vi "re_DataLog Query_srv.vi"(0 "method":T3, 1 "time step":dbl, 5 "begin of range":dbl format="%<%H:%M:%S%2u\n%Y/%m/%d>T", 7 "certificate":string, 9 "end of range":dbl format="%<%H:%M:%S%2u\n%Y/%m/%d>T", 11 "tag":string, 12 "database (current)":string) -> (3 "mode {read range}":T1, 4 "values":dbl[](array[numeric]), 6 "times":dbl[](array[numeric]) format="%<%H:%M:%S%2u\n%Y/%m/%d>T", 8 "points":T2[](array[typedef]) {"value" format="%.3e"; "time" format="%<%H:%M:%S%2u\n%Y/%m/%d>T"}, 10 "strings":string[](array[string]), 15 "error out":errorcluster)   [LabVIEW 2012]
uses:
  typedefs/t_DataLog Query Served Methods.ctl
  typedefs/t_Datalog Datebase Modes.ctl
  typedefs/clusters/t_DataLog Point.ctl
  clientsrv/typedefs/t_ClientSrv Access Levels.ctl
  typedefs/t_DataLog Databases Methods.ctl
  typedefs/t_DataLog Tag Info List Methods.ctl
  subvis/private/glb_DataLog Runtime Parameterisation.vi
panel:
  # "Update panel typedef\nafter changing panel."
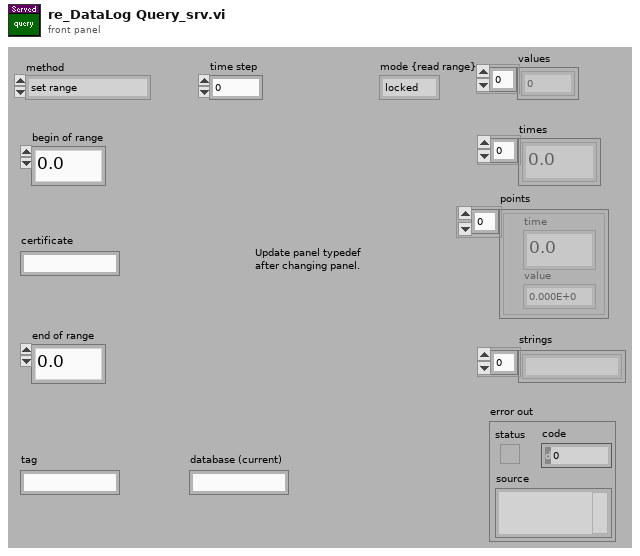
[diagram p1: front panel]
types:
  T1 = typedef "t_Datalog Datebase Modes.ctl" = enum16{"locked", "unlocked", "live", "mirrored"}
  T2 = typedef "t_DataLog Point.ctl" = cluster{"time":dbl, "value":dbl}
  T3 = typedef "t_DataLog Query Served Methods.ctl" = enum16{"set range", "step times", "get times", "interpolate", "interpolate str", "read range", "read str range", "merge&read range", "merge&read str range", "merge range", "clear"}
  T4 = typedef "t_ClientSrv Access Levels.ctl" = enum16{"observer", "operator", "local"}
  T5 = typedef "t_DataLog Tag Info List Methods.ctl" = enum16{"initialize", "create", "create empty", "rename", "delete", "test tag", "get", "get by name", "get default", "get list", "get path", "get subsets", "set subsets", "set config", "set capacity", "#tags", "go live", "set unlocked", "set mirrored"}
  T6 = typedef "t_DataLog Databases Methods.ctl" = enum16{"initialize", "get ref", "get names", "cleanup"}
  T7 = typedef "t_DataLog Database Info Pane.ctl" = refnum<vi>
  T8 = typedef "t_DataLog Tag Config.ctl" = cluster{"name":string, "unit":string, "temporal":T9, "value":T10, "index":i32, "capacity":i32, "is meta?":bool, "mincapacity":i32, "deadband":dbl, "limit delay":dbl, "format":T11, "precision":u8, "undefine":bool, "update":bool, "update period":u16, "expression":string, "description":string, "logging algorithm":T12, "logging parameters":dbl[]}
  T9 = typedef "t_DataLog Temporal Types.ctl" = enum16{"set&hold", "sample", "event"}
  T10 = typedef "t_DataLog Value Types.ctl" = enum16{"number", "string"}
  T11 = typedef "t_DataLog Numerical Format.ctl" = enum8{"fractional", "exponential", "engineering"}
  T12 = typedef "t_DataLog Logging Algorithms.ctl" = enum16{"nothing", "changes", "everything", "every Nth", "time threshold", "value threshold + prior", "t or v threshold", "t or v threshold + prior"}
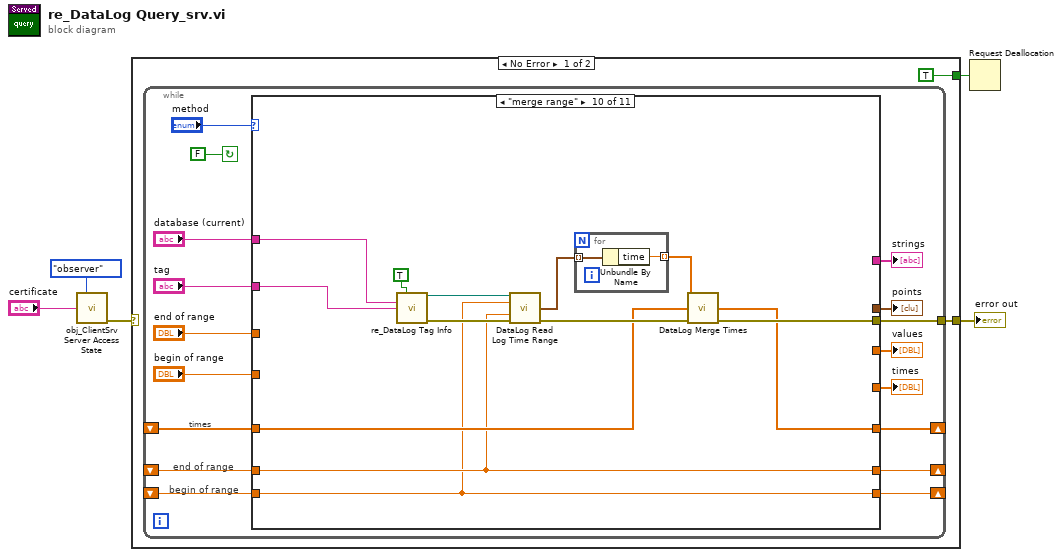
[diagram p0: block diagram]
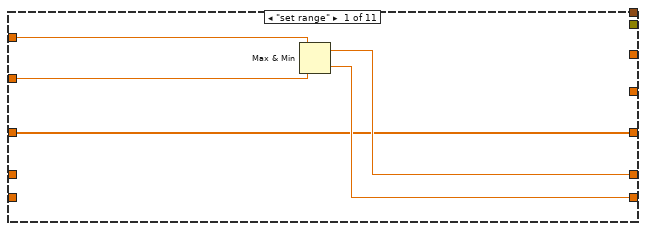
[diagram p2: hidden frame]
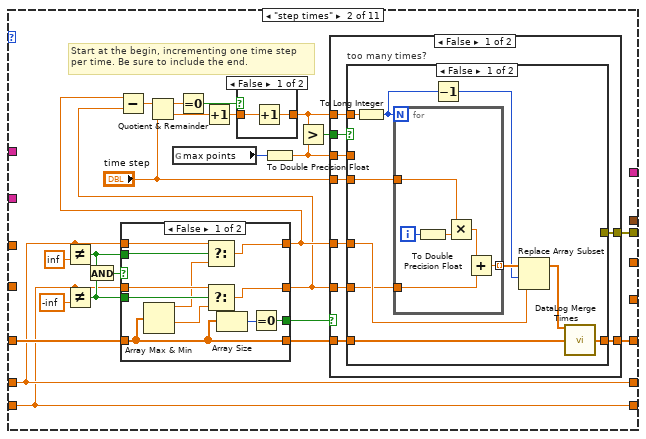
[diagram p3: hidden frame]
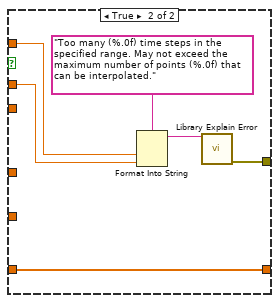
[diagram p4: hidden frame]
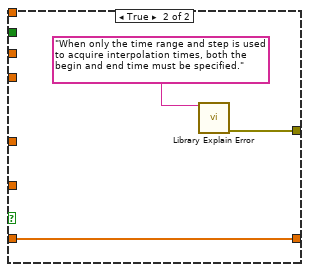
[diagram p5: hidden frame]
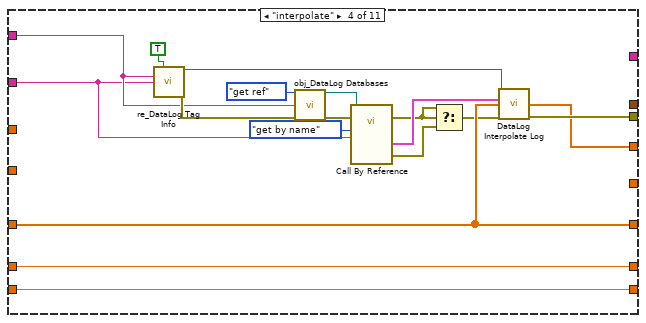
[diagram p9: hidden frame]
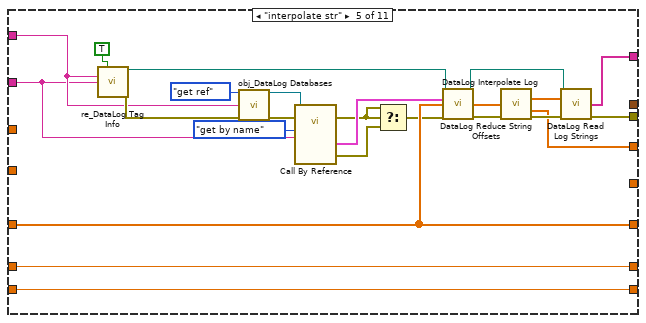
[diagram p10: hidden frame]
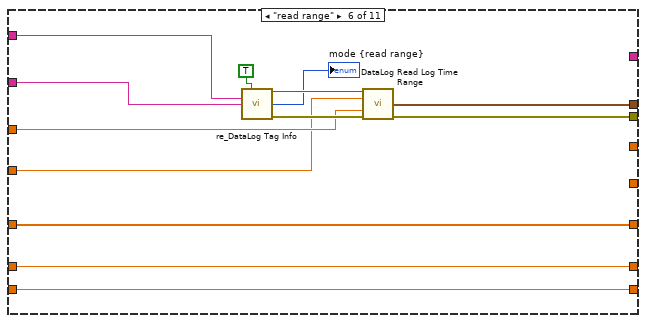
[diagram p11: hidden frame]
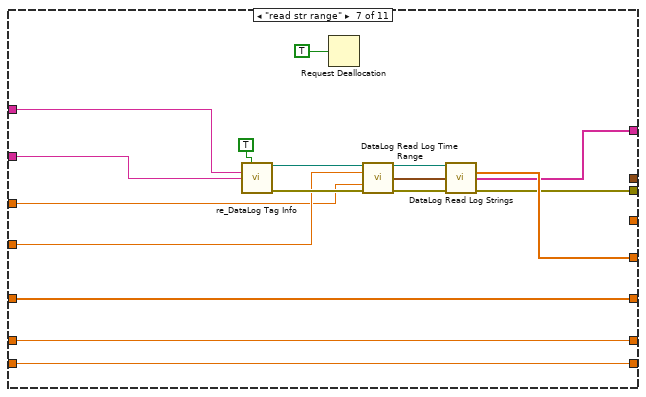
[diagram p12: hidden frame]
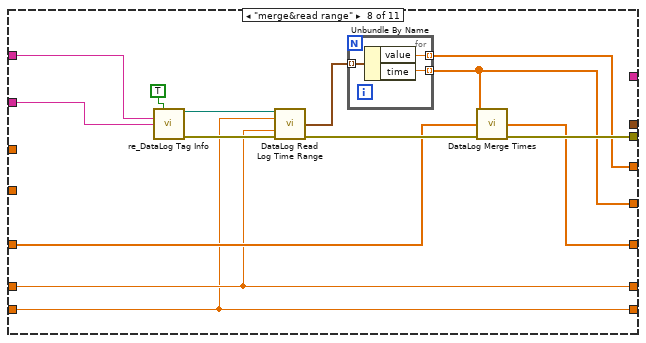
[diagram p13: hidden frame]
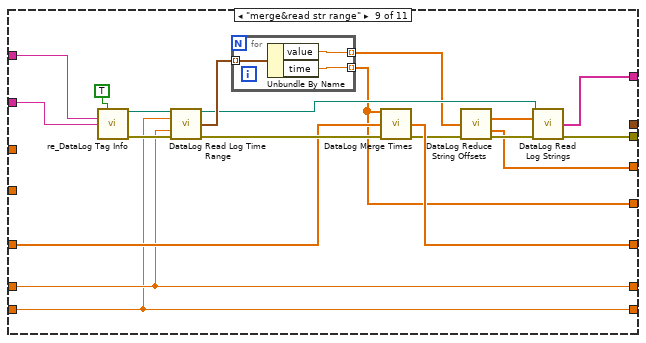
[diagram p14: hidden frame]
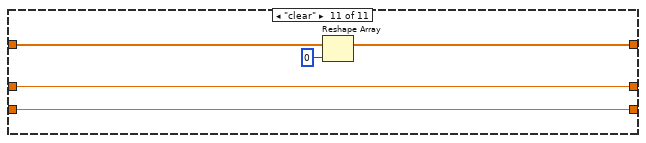
[diagram p15: hidden frame]
diagram:
  n1 = call "obj_ClientSrv Server Access State.vi"("access level"=t_ClientSrv_Access_Levels."observer", "certificate in"="certificate") -> ("error out"=w2:errorcluster)  [unwired: 11 in, 2 out]
  n2 = case shown="No Error" w2 {
    selector: w2 -> [_ w240]
    tunnel: [w7 w240] -> w3
    tunnel: [TRUE ("flag") _] -> w1
    frame No Error {
      n3 = while {
        shift-right: [w18] -> _
        shift-left: _ -> [w19]
        tunnel: [w17] -> w7
        shift-right: [w12] -> _
        shift-left: _ -> [w11]
        shift-right: [w9] -> _
        shift-left: _ -> [w10]
        stop <- FALSE continue-if-true
        # "begin of range"
        # "end of range"
        # "times"
        n4 = case shown="\"merge range\"" "method" {
          tunnel: "begin of range" -> [w28 _ _ _ _ w151 w165 _ _ _ _]
          tunnel: "end of range" -> [w29 _ _ _ _ w153 w163 _ _ _ _]
          tunnel: "tag" -> [_ _ _ w114 w140 w162 w179 w193 w216 w232 _]
          tunnel: w19 -> [w25 w39 w107 w122 w147 w155 w174 w186 w210 w225 w239]
          tunnel: [w25 w43 w107 w122 w147 w155 w174 w185 w209 w224 w238] -> w18
          tunnel: [_ w46 _ w123 w131 w157 w168 w187 w205 w226 _] -> w17
          tunnel: [_ _ w107 _ _ _ w171 w181 w198 _ _] -> w16
          tunnel: "database (current)" -> [_ _ _ w119 w145 w160 w177 w191 w214 w230 _]
          tunnel: [_ _ _ w121 w126 _ _ w180 w199 _ _] -> w14
          tunnel: [_ _ _ _ _ w156 _ _ _ _ _] -> w13
          tunnel: [w27 w36 w106 w109 w135 w154 w164 w184 w208 w223 w236] -> w12
          tunnel: w11 -> [_ w36 w106 w109 w135 w154 w164 w184 w208 w223 w236]
          tunnel: w10 -> [_ w33 w105 w108 w134 w152 w166 w183 w207 w222 w235]
          tunnel: [w26 w33 w105 w108 w134 w152 w166 w183 w207 w222 w235] -> w9
          tunnel: [_ _ _ _ w132 _ w170 _ w206 _ _] -> w8
          frame "set range" {
            n5 = Max & Min(x=w29, y=w28) -> (max(x,y)=w27:dbl, min(x,y)=w26:dbl)
          }
          frame "step times" {
            # "Start at the begin, incrementing one time step\nper time. Be sure to include the end."
            n6 = Not Equal?(x=w36, y=inf) -> (x != y?=w35:bool)
            n7 = Not Equal?(x=w33, y=-inf) -> (x != y?=w34:bool)
            n8 = And(x=w35, y=w34) -> (x .and. y?=w38:bool)
            n9 = case shown="False" w38 {
              tunnel: w39 -> [w90 w101]
              tunnel: [w90 w101] -> w37
              tunnel: w36 -> [w95 w99]
              tunnel: w35 -> [w92 _]
              tunnel: w34 -> [w97 _]
              tunnel: w33 -> [w98 w100]
              tunnel: [w94 w100] -> w31
              tunnel: [w93 w99] -> w32
              tunnel: [w88 _] -> w30
              frame False {
                n10 = Array Max & Min(array=w90) -> (max value=w91:dbl, min value=w96:dbl)  [unwired: 2 out]
                n11 = Select(t=w95, s=w92, f=w91) -> (s? t:f=w93:dbl)
                n12 = Select(t=w98, s=w97, f=w96) -> (s? t:f=w94:dbl)
                n13 = Array Size(array=w90) -> (size(s)=w89:i32)
                n14 = Equal To 0?(x=w89) -> (x = 0?=w88:bool)
              }
              frame True {
              }
            }
            n15 = Subtract(x=w32, y=w31) -> (x-y=w53:dbl)
            n16 = Quotient & Remainder(x=w53, y="time step") -> (x-y*floor(x/y)=w52:dbl, floor(x/y)=w51:dbl)
            n17 = global read "glb_DataLog Runtime Parameterisation.vi" "max points"() -> (w48:i32)
            n18 = Equal To 0?(x=w52) -> (x = 0?=w50:bool)
            n19 = Increment(x=w51) -> (x+1=w49:dbl)
            n20 = case shown="False" w50 {
              tunnel: w49 -> [w103 w104]
              tunnel: [w102 w104] -> w44
              frame False {
                n21 = Increment(x=w103) -> (x+1=w102:dbl)
              }
              frame True {
              }
            }
            n22 = To Double Precision Float(number=w48) -> (double precision float=w45:dbl)
            n23 = Greater?(x=w44, y=w45) -> (0:w47:bool)
            n24 = case shown="False" w30 {
              tunnel: w47 -> [w62 _]
              tunnel: [w61 w86] -> w46
              tunnel: w45 -> [w60 _]
              tunnel: w44 -> [w59 _]
              tunnel: [w58 w85] -> w43
              tunnel: "time step" -> [w57 _]
              tunnel: w37 -> [w56 w85]
              tunnel: w32 -> [w55 _]
              tunnel: w31 -> [w54 _]
              frame False {
                n25 = case "too many times?" shown="False" w62 {
                  tunnel: [_ w83] -> w61
                  tunnel: w60 -> [_ w80]
                  tunnel: w59 -> [w72 w81]
                  tunnel: w57 -> [w71 _]
                  tunnel: [w67 w79] -> w58
                  tunnel: w56 -> [w65 w79]
                  tunnel: w55 -> [w64 _]
                  tunnel: w54 -> [w63 _]
                  frame False {
                    n26 = To Long Integer(number=w72) -> (32bit integer=w69:i32)
                    n27 = for {
                      N: w69 -> [_]
                      tunnel: w71 -> [w78]
                      tunnel: [w74] -> w70 mode=indexing
                      tunnel: w63 -> [w73]
                      i -> [w77]
                      n28 = To Double Precision Float(number=w77) -> (double precision float=w76:dbl)
                      n29 = Multiply(x=w78, y=w76) -> (x*y=w75:dbl)
                      n30 = Add(x=w75, y=w73) -> (x+y=w74:dbl)
                    }
                    n31 = Decrement(x=w69) -> (x-1=w68:i32)
                    n32 = Replace Array Subset(array=w70, new element=w64, index=w68) -> (w66:dbl[])
                    n33 = call "DataLog Merge Times.vi"("times to add"=w66, "times in"=w65) -> ("times out"=w67:dbl[])  [unwired: 12 in, 1 out]
                  }
                  frame True {
                    n34 = Format Into String(format string="Too many (%.0f) time steps in the specified range. May not exceed the maximum number of points (%.0f) that can be interpolated.", w81, w80) -> (resulting string=w82:string)  [unwired: 2 in, 1 out]
                    n35 = call "Library Explain Error.vi"("explanation prefix (none)"=w82) -> ("explained error"=w83:errorcluster)  [unwired: 14 in]
                  }
                }
              }
              frame True {
                n36 = call "Library Explain Error.vi"("explanation prefix (none)"="When only the time range and step is used to acquire interpolation times, both the begin and end time must be specified." ("format string")) -> ("explained error"=w86:errorcluster)  [unwired: 14 in]
              }
            }
          }
          frame "get times" {
          }
          frame "interpolate" {
            n37 = call "re_DataLog Tag Info.vi"("flush? (false)"=TRUE, "database (current)"=w119, "tag"=w114) -> ("tag log directory"=w124:path, "error out"=w120:errorcluster)  [unwired: 9 in, 2 out]
            n38 = call "obj_DataLog Databases.vi"("method"=t_DataLog_Databases_Methods."get ref", "database (current)"=w119, "error in (no error)"=w120) -> ("database ref"=w116:T7, "error out"=w117:errorcluster)  [unwired: 10 in, 1 out]
            n39 = call-by-ref "?"(reference=w116, error in=w117, "method"=t_DataLog_Tag_Info_List_Methods."get by name", "tag or base tag"=w114) -> (error out=w112:errorcluster, "tag config out"=w113:T8, 15:"error out"=w111:errorcluster)  [unwired: 7 in, 6 out]
            n40 = Select(t=w112, s=w112, f=w111) -> (s? t:f=w110:errorcluster)
            n41 = call "DataLog Interpolate Log.vi"("tag log directory"=w124, "tag config"=w113, "times"=w122, "error in (no error)"=w110) -> ("interpolated values"=w121:dbl[], "error out"=w123:errorcluster)  [unwired: 8 in, 2 out]
          }
          frame "interpolate str" {
            n42 = call "re_DataLog Tag Info.vi"("flush? (false)"=TRUE, "database (current)"=w145, "tag"=w140) -> ("tag log directory"=w148:path, "error out"=w146:errorcluster)  [unwired: 9 in, 2 out]
            n43 = call "obj_DataLog Databases.vi"("method"=t_DataLog_Databases_Methods."get ref", "database (current)"=w145, "error in (no error)"=w146) -> ("database ref"=w142:T7, "error out"=w143:errorcluster)  [unwired: 10 in, 1 out]
            n44 = call-by-ref "?"(reference=w142, error in=w143, "method"=t_DataLog_Tag_Info_List_Methods."get by name", "tag or base tag"=w140) -> (error out=w138:errorcluster, "tag config out"=w139:T8, 15:"error out"=w137:errorcluster)  [unwired: 7 in, 6 out]
            n45 = Select(t=w138, s=w138, f=w137) -> (s? t:f=w136:errorcluster)
            n46 = call "DataLog Interpolate Log.vi"("tag log directory"=w148, "tag config"=w139, "times"=w147, "error in (no error)"=w136) -> ("dup tag log directory"=w133:path, "interpolated values"=w129:dbl[], "error out"=w130:errorcluster)  [unwired: 8 in, 1 out]
            n47 = call "DataLog Reduce String Offsets.vi"("string offsets"=w129, "error in (no error)"=w130) -> ("reduced offsets"=w128:dbl[], "string indices"=w126:dbl[], "error out"=w127:errorcluster)  [unwired: 11 in]
            n48 = call "DataLog Read Log Strings.vi"("tag log directory"=w133, "offsets (use points)"=w128, "error in (no error)"=w127) -> ("strings"=w132:string[], "error out"=w131:errorcluster)  [unwired: 9 in, 2 out]
          }
          frame "read range" {
            n49 = call "re_DataLog Tag Info.vi"("flush? (false)"=TRUE, "database (current)"=w160, "tag"=w162) -> ("tag log directory"=w159:path, "mode"=→"mode {read range}":T1, "error out"=w158:errorcluster)  [unwired: 9 in, 1 out]
            n50 = call "DataLog Read Log Time Range.vi"("tag log directory"=w159, "begin of range"=w151, "end of range"=w153, "error in (no error)"=w158) -> ("time range of points"=w156:T2[], "error out"=w157:errorcluster)  [unwired: 8 in, 2 out]
          }
          frame "read str range" {
            n51 = call "re_DataLog Tag Info.vi"("flush? (false)"=TRUE, "database (current)"=w177, "tag"=w179) -> ("tag log directory"=w176:path, "error out"=w175:errorcluster)  [unwired: 9 in, 2 out]
            n52 = Request Deallocation(TRUE ("flag")) -> ()
            n53 = call "DataLog Read Log Time Range.vi"("tag log directory"=w176, "begin of range"=w165, "end of range"=w163, "error in (no error)"=w175) -> ("dup tag log directory"=w169:path, "time range of points"=w173:T2[], "error out"=w172:errorcluster)  [unwired: 8 in, 1 out]
            n54 = call "DataLog Read Log Strings.vi"("tag log directory"=w169, "points (use offsets)"=w173, "error in (no error)"=w172) -> ("times"=w171:dbl[], "strings"=w170:string[], "error out"=w168:errorcluster)  [unwired: 9 in, 1 out]
          }
          frame "merge&read range" {
            n55 = call "re_DataLog Tag Info.vi"("flush? (false)"=TRUE, "database (current)"=w191, "tag"=w193) -> ("tag log directory"=w190:path, "error out"=w189:errorcluster)  [unwired: 9 in, 2 out]
            n56 = call "DataLog Read Log Time Range.vi"("tag log directory"=w190, "begin of range"=w183, "end of range"=w184, "error in (no error)"=w189) -> ("time range of points"=w182:T2[], "error out"=w188:errorcluster)  [unwired: 8 in, 2 out]
            n57 = for {
              tunnel: w182 -> [w196] mode=indexing
              tunnel: [w195] -> w181 mode=indexing
              tunnel: [w194] -> w180 mode=indexing
              n58 = Unbundle By Name(w196) -> ("value"=w194:dbl, "time"=w195:dbl)
            }
            n59 = call "DataLog Merge Times.vi"("times to add"=w181, "times in"=w186, "error in (no error)"=w188) -> ("times out"=w185:dbl[], "error out"=w187:errorcluster)  [unwired: 11 in]
          }
          frame "merge&read str range" {
            n60 = call "re_DataLog Tag Info.vi"("flush? (false)"=TRUE, "database (current)"=w214, "tag"=w216) -> ("tag log directory"=w213:path, "error out"=w212:errorcluster)  [unwired: 9 in, 2 out]
            n61 = call "DataLog Read Log Time Range.vi"("tag log directory"=w213, "begin of range"=w207, "end of range"=w208, "error in (no error)"=w212) -> ("dup tag log directory"=w201:path, "time range of points"=w204:T2[], "error out"=w211:errorcluster)  [unwired: 8 in, 1 out]
            n62 = for {
              tunnel: w204 -> [w219] mode=indexing
              tunnel: [w218] -> w198 mode=indexing
              tunnel: [w217] -> w200 mode=indexing
              n63 = Unbundle By Name(w219) -> ("value"=w217:dbl, "time"=w218:dbl)
            }
            n64 = call "DataLog Merge Times.vi"("times to add"=w198, "times in"=w210, "error in (no error)"=w211) -> ("times out"=w209:dbl[], "error out"=w203:errorcluster)  [unwired: 11 in]
            n65 = call "DataLog Reduce String Offsets.vi"("string offsets"=w200, "error in (no error)"=w203) -> ("reduced offsets"=w197:dbl[], "string indices"=w199:dbl[], "error out"=w202:errorcluster)  [unwired: 11 in]
            n66 = call "DataLog Read Log Strings.vi"("tag log directory"=w201, "offsets (use points)"=w197, "error in (no error)"=w202) -> ("strings"=w206:string[], "error out"=w205:errorcluster)  [unwired: 9 in, 2 out]
          }
          frame "merge range" {
            n67 = call "re_DataLog Tag Info.vi"("flush? (false)"=TRUE, "database (current)"=w230, "tag"=w232) -> ("tag log directory"=w229:path, "error out"=w228:errorcluster)  [unwired: 9 in, 2 out]
            n68 = call "DataLog Read Log Time Range.vi"("tag log directory"=w229, "begin of range"=w222, "end of range"=w223, "error in (no error)"=w228) -> ("time range of points"=w221:T2[], "error out"=w227:errorcluster)  [unwired: 8 in, 2 out]
            n69 = for {
              tunnel: w221 -> [w234] mode=indexing
              tunnel: [w233] -> w220 mode=indexing
              n70 = Unbundle By Name(w234) -> ("time"=w233:dbl)
            }
            n71 = call "DataLog Merge Times.vi"("times to add"=w220, "times in"=w225, "error in (no error)"=w227) -> ("times out"=w224:dbl[], "error out"=w226:errorcluster)  [unwired: 11 in]
          }
          frame "clear" {
            n72 = Reshape Array(w239, 0 ("dimension size")) -> (w238:dbl[])
          }
        }
        "times" <- w16
        "values" <- w14
        "points" <- w13
        "strings" <- w8
      }
    }
    frame Error {
    }
  }
  "error out" <- w3
  n73 = Request Deallocation(w1) -> ()
